vi "Error Handler.vi"(8 "error in (no error)":errorcluster, 10 "state":T1=enum."Start", 11 "Plugin Thread in":refnum<class "Plugin Thread.lvclass">) -> (0 "error out":errorcluster, 3 "Plugin Thread out":refnum<class "Plugin Thread.lvclass">)   [LabVIEW 2017, in "DSF Core.lvlib" / "Plugin Thread.lvclass"]
uses:
  Thread/Plugin/Plugin Thread.lvclass
  C:/Git/DSF/Core/Classes/Thread/Thread.lvclass
  Interface/Plugin/Command.ctl
  Thread/Thread.lvclass
  Interface/Plugin/Plugin Interface.lvclass
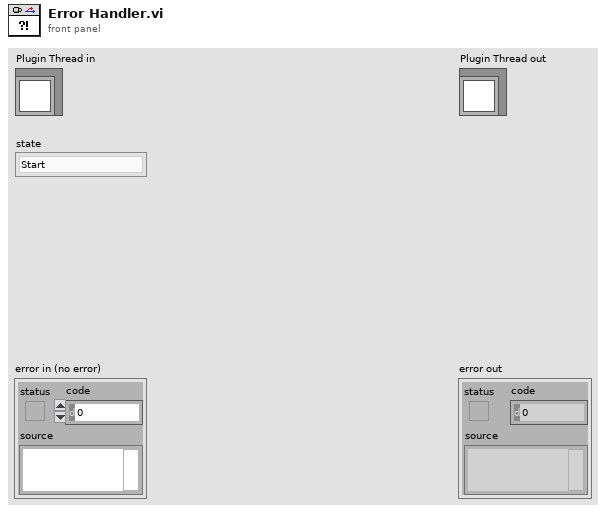
[diagram p1: front panel]
types:
  T1 = typedef "DSF Core.lvlib/Plugin Interface.lvclass/Command.ctl" = enum8{"Idle", "Start", "Set Inline Buffer", "Rx", "Tx", "Shutdown", "Error"}
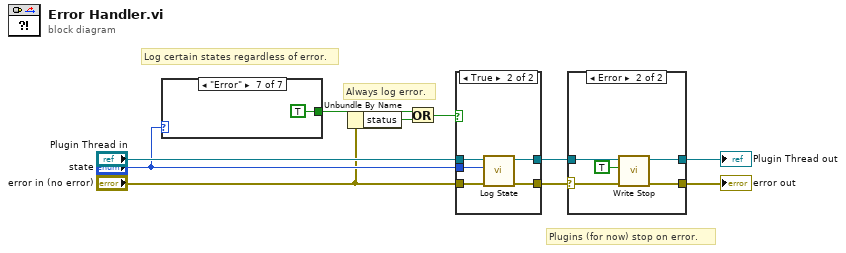
[diagram p0: block diagram]
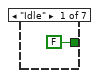
[diagram p2: hidden frame]
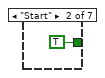
[diagram p3: hidden frame]
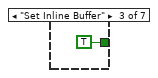
[diagram p4: hidden frame]
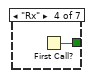
[diagram p5: hidden frame]
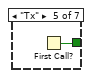
[diagram p6: hidden frame]
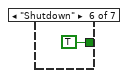
[diagram p7: hidden frame]
diagram:
  # "Plugins (for now) stop on error."
  # "Log certain states regardless of error."
  # "Always log error."
  n1 = case shown="\"Error\"" "state" {
    tunnel: [FALSE ("First Call?: T/F") TRUE TRUE ("status") w14 w15 TRUE ("First Call?: T/F") TRUE ("First Call?: T/F")] -> w9
    frame "Idle" {
    }
    frame "Start" {
    }
    frame "Set Inline Buffer" {
    }
    frame "Rx" {
      n2 = First Call?() -> (First Call?: T/F=w14:bool)
    }
    frame "Tx" {
      n3 = First Call?() -> (First Call?: T/F=w15:bool)
    }
    frame "Shutdown" {
    }
    frame "Error" {
    }
  }
  n4 = Unbundle By Name("error in (no error)") -> ("status"=w8:bool)
  n5 = Or(x=w9, y=w8) -> (x .or. y?=w7:bool)
  n6 = case shown="True" w7 {
    tunnel: [w19 w21] -> w3
    tunnel: [w18 w20] -> w4
    tunnel: "Plugin Thread in" -> [w19 w24]
    tunnel: "error in (no error)" -> [w18 w23]
    tunnel: "state" -> [_ w22]
    frame False {
    }
    frame True {
      n7 = call "Log State.vi"("error in (no error)"=w23, "state"=w22, "Plugin Thread in"=w24) -> ("error out"=w20:errorcluster, "Plugin Thread out"=w21:refnum<class "Plugin Thread.lvclass">)  [unwired: 7 in]
    }
  }
  n8 = case shown="Error" w4 {
    selector: w4 -> [w26 w30]
    tunnel: w3 -> [w25 w29]
    tunnel: [w26 w27] -> w2
    tunnel: [w25 w28] -> w1
    frame No Error {
    }
    frame Error {
      n9 = call "Write Stop.vi"("error in (no error)"=w30, "stop"=TRUE, "Thread in"=w29) -> ("error out"=w27:errorcluster, "Thread out"=w28:refnum<class "Plugin Thread.lvclass">)  [unwired: 7 in]
    }
  }
  "error out" <- w2
  "Plugin Thread out" <- w1
